vi "GetDeviceInfo.vi"(8 "error in (no error)":errorcluster, 11 "DAQSuper in":refnum<class "DAQSuper.lvclass">) -> (0 "error out":errorcluster, 1 "MaxSampleClock":dbl, 2 "ChannelCount":dbl, 3 "DAQSuper out":refnum<class "DAQSuper.lvclass">, 5 "DeviceName":string)   [LabVIEW 2013, in "DAQSuper.lvclass"]
uses:
  DAQSuper.lvclass
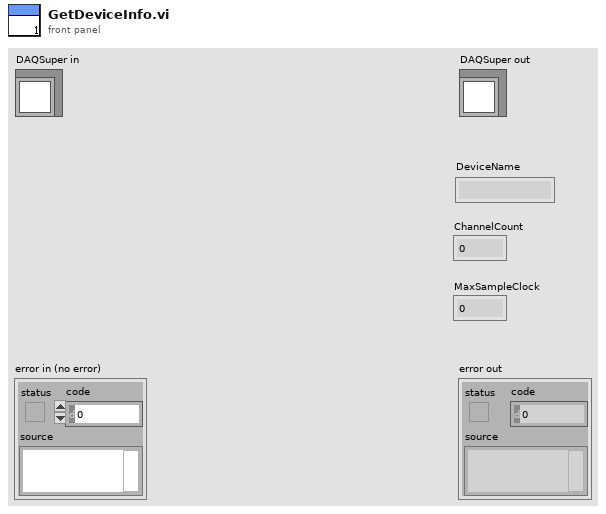
[diagram p1: front panel]
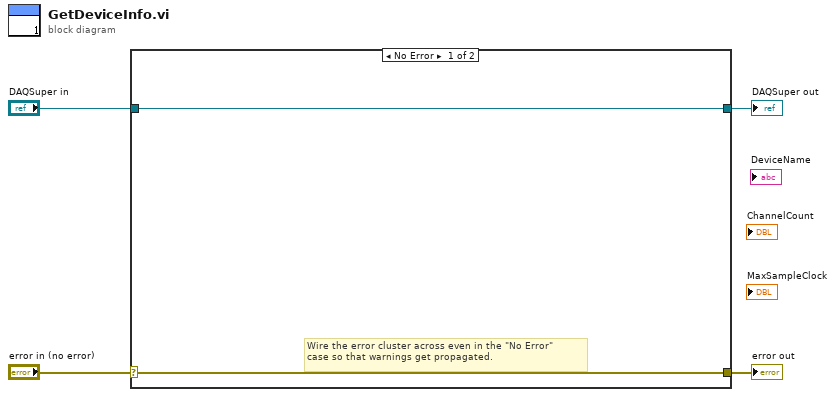
[diagram p0: block diagram]
diagram:
  n1 = case shown="No Error" "error in (no error)" {
    selector: "error in (no error)" -> [w5 w8]
    tunnel: [w5 w8] -> w3
    tunnel: [w6 w7] -> w1
    tunnel: "DAQSuper in" -> [w6 w7]
    frame No Error {
      # "Wire the error cluster across even in the \"No Error\"\ncase so that warnings get propagated."
    }
    frame Error {
    }
  }
  "error out" <- w3
  "DAQSuper out" <- w1
